vi "NCC Setup Results Array - U16.vi"(0 "Image 01 Size":i32[](array[numeric]), 2 "Half Shift":i32, 11 "Image 02 Size":i32[](array[numeric])) -> (4 "NCC Results Array":dbl[](array[numeric]), 8 "Result Rows":i32, 15 "Result Columns":i32)   [LabVIEW 2020]
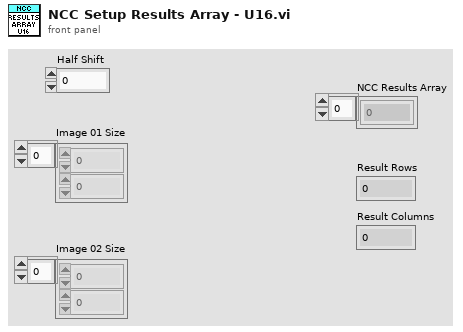
[diagram p1: front panel]
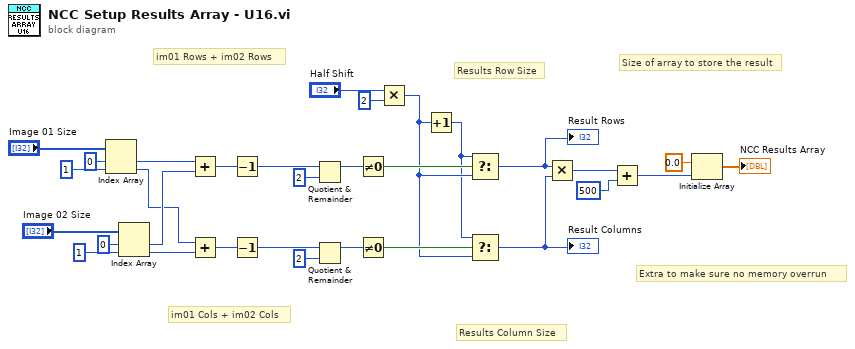
[diagram p0: block diagram]
diagram:
  # "im01 Cols + im02 Cols"
  # "im01 Rows + im02 Rows"
  # "Extra to make sure no memory overrun"
  # "Size of array to store the result"
  # "Results Column Size"
  # "Results Row Size"
  n1 = Index Array(array="Image 01 Size", index #1=0 ("index"), index #2=1 ("index")) -> (element #1=w4:i32, element #2=w1:i32)
  n2 = Index Array(array="Image 02 Size", index #1=0 ("index"), index #2=1 ("index")) -> (element #1=w3:i32, element #2=w2:i32)
  n3 = Add(x=w4, y=w3) -> (x+y=w31:i32)
  n4 = Add(x=w1, y=w2) -> (x+y=w24:i32)
  n5 = Decrement(x=w31) -> (x-1=w30:i32)
  n6 = Decrement(x=w24) -> (x-1=w23:i32)
  n7 = Quotient & Remainder(x=w30, y=2) -> (x-y*floor(x/y)=w28:i32)  [unwired: 1 out]
  n8 = Quotient & Remainder(x=w23, y=2) -> (x-y*floor(x/y)=w21:i32)  [unwired: 1 out]
  n9 = Not Equal To 0?(x=w28) -> (x != 0?=w27:bool)
  n10 = Not Equal To 0?(x=w21) -> (x != 0?=w20:bool)
  n11 = Multiply(x="Half Shift", y=2) -> (x*y=w19:i32)
  n12 = Increment(x=w19) -> (x+1=w18:i32)
  n13 = Select(t=w18, s=w27, f=w19) -> (s? t:f=w17:i32)
  "Result Rows" <- w17
  n14 = Select(t=w18, s=w20, f=w19) -> (s? t:f=w16:i32)
  "Result Columns" <- w16
  n15 = Multiply(x=w17, y=w16) -> (x*y=w15:i32)
  n16 = Add(x=w15, y=500) -> (x+y=w13:i32)
  n17 = Initialize Array(0.0 ("element"), w13) -> (→"NCC Results Array":dbl[])
